vi "Untitled 1.vi"() -> ()   [LabVIEW 2023]
panel:
  out "Signals":dynamicdata(graph)
  out "Waveform Graph":dbl[](graph)
  out "size(s)":i32=4
  in  "Filename":path=path "D:/Mega/CyA/AypProgs/Programas Chips Ingeniería/Arduino/Labview cedim/totalcode/data11.lvm"
  out "Signals 2":dbl=20.0
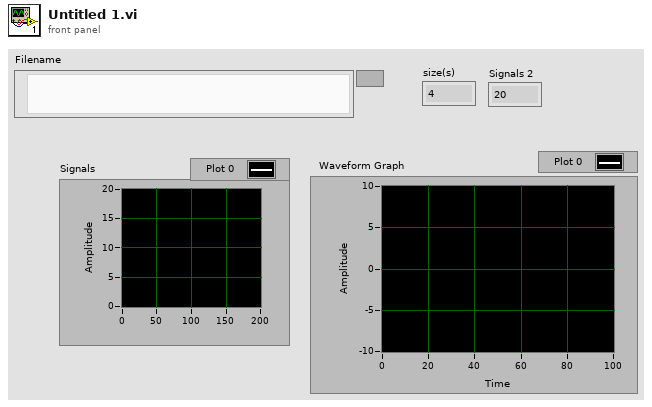
[diagram p1: front panel]
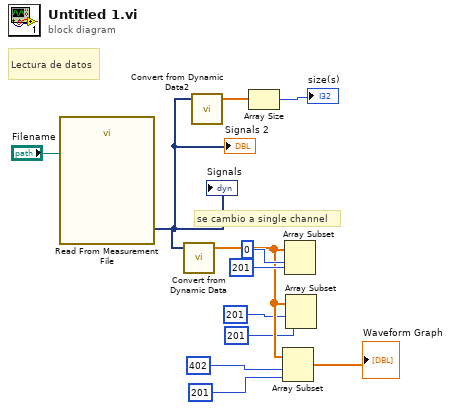
[diagram p0: block diagram]
diagram:
  # "se cambio a single channel"
  # "Lectura de datos"
  n1 = call "Read From Measurement File"("Filename"="Filename") -> ("Signals"=w7:dynamicdata)  [unwired: 5 in, 5 out]
  "Signals 2" <- w7
  "Signals" <- w7
  n2 = call "Convert from Dynamic Data"("Dynamic Data Type"=w7) -> ("Array"=w6:dbl[])  [unwired: 3 in]
  n3 = call "Convert from Dynamic Data2"("Dynamic Data Type"=w7) -> ("Array"=w11:dbl[])  [unwired: 3 in]
  n4 = Array Size(array=w11) -> (size(s)=→"size(s)":i32)
  n5 = Array Subset(array=w6, index=402, length=201) -> (→"Waveform Graph":dbl[])
  n6 = Array Subset(array=w6, index=0, length=201) -> ()  [unwired: 1 out]
  n7 = Array Subset(array=w6, index=201, length=201) -> ()  [unwired: 1 out]
